vi "Hatch Manipulator Controller.vi"(8 "error in":errorcluster) -> ()   [LabVIEW 2018]
doc: "This VI executes continuously carrying out the current operation and responding to updates or new operations. It will often contain the timing or control code that is difficult to place directly in TeleOp. This VI generally opens all sensors and motors and isolates the rest of the robot code from knowing how the operations are carried out."
uses:
  Hatch Manipulator Setpoints.ctl
  Hatch Manipulator Operations.ctl
  <vilib>/Rock Robotics/WPI/Solenoid/WPI_SolenoidChannel.ctl
  <vilib>/Rock Robotics/WPI/Solenoid/WPI_SolenoidValue.ctl
  <vilib>/Rock Robotics/WPI/Solenoid/WPI_SolenoidOpenSingle.vi
  <vilib>/Rock Robotics/WPI/Solenoid/WPI_SolenoidSetEnum.vi
panel:
  out "Current\nCmd":string
  # "Tip: It may be helpful to observe inputs and sensor values.\nYou may also want to display tuning or debugging controls."
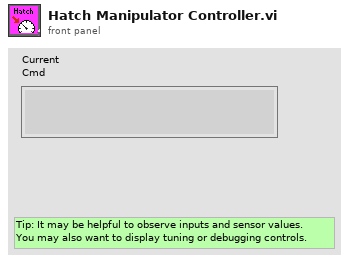
[diagram p1: front panel]
types:
  T1 = typedef "WPI_SolenoidValue.ctl" = enum16{"Off", "On", "Forward", "Reverse"}
  T2 = typedef "WPI_SolenoidChannel.ctl" = enum8{"Solenoid 0", "Solenoid 1", "Solenoid 2", "Solenoid 3", "Solenoid 4", "Solenoid 5", "Solenoid 6", "Solenoid 7", "Invalid"}
  T3 = typedef "Hatch Manipulator Setpoints.ctl" = cluster{"Operation":T4, "Setpoint":dbl, "Duration":dbl}
  T4 = typedef "Hatch Manipulator Operations.ctl" = enum16{"Reserve", "Read Current", "Immediate", "Out", "In", "Open", "Close"}
  T5 = typedef "WPI_SolenoidDevRef.ctl" = cluster{"DevStatus":errorcluster, "Pneumatics Control Module":u8, "Forward Solenoid Channel":T2, "Reverse Solenoid Channel":T2}
  T6 = typedef "Command Status Info.ctl" = cluster{"Name":string, "Status":T7, "notifier out":T8}
  T7 = typedef "Completion Status.ctl" = enum16{"Successful", "Aborted", "Incomplete"}
  T8 = typedef "Completion Notifier.ctl" = refnum<notifier>
  T9 = cluster{"Current Command":T3, "Command Timing":cluster{"Start Time (ms)":u32, "Iterations":i32}, "Command Arguments":cluster{"Command Info":T6, "Description":string, "Default Command":T3, "queue out":refnum<queue>, "Subsystem Name":string}}
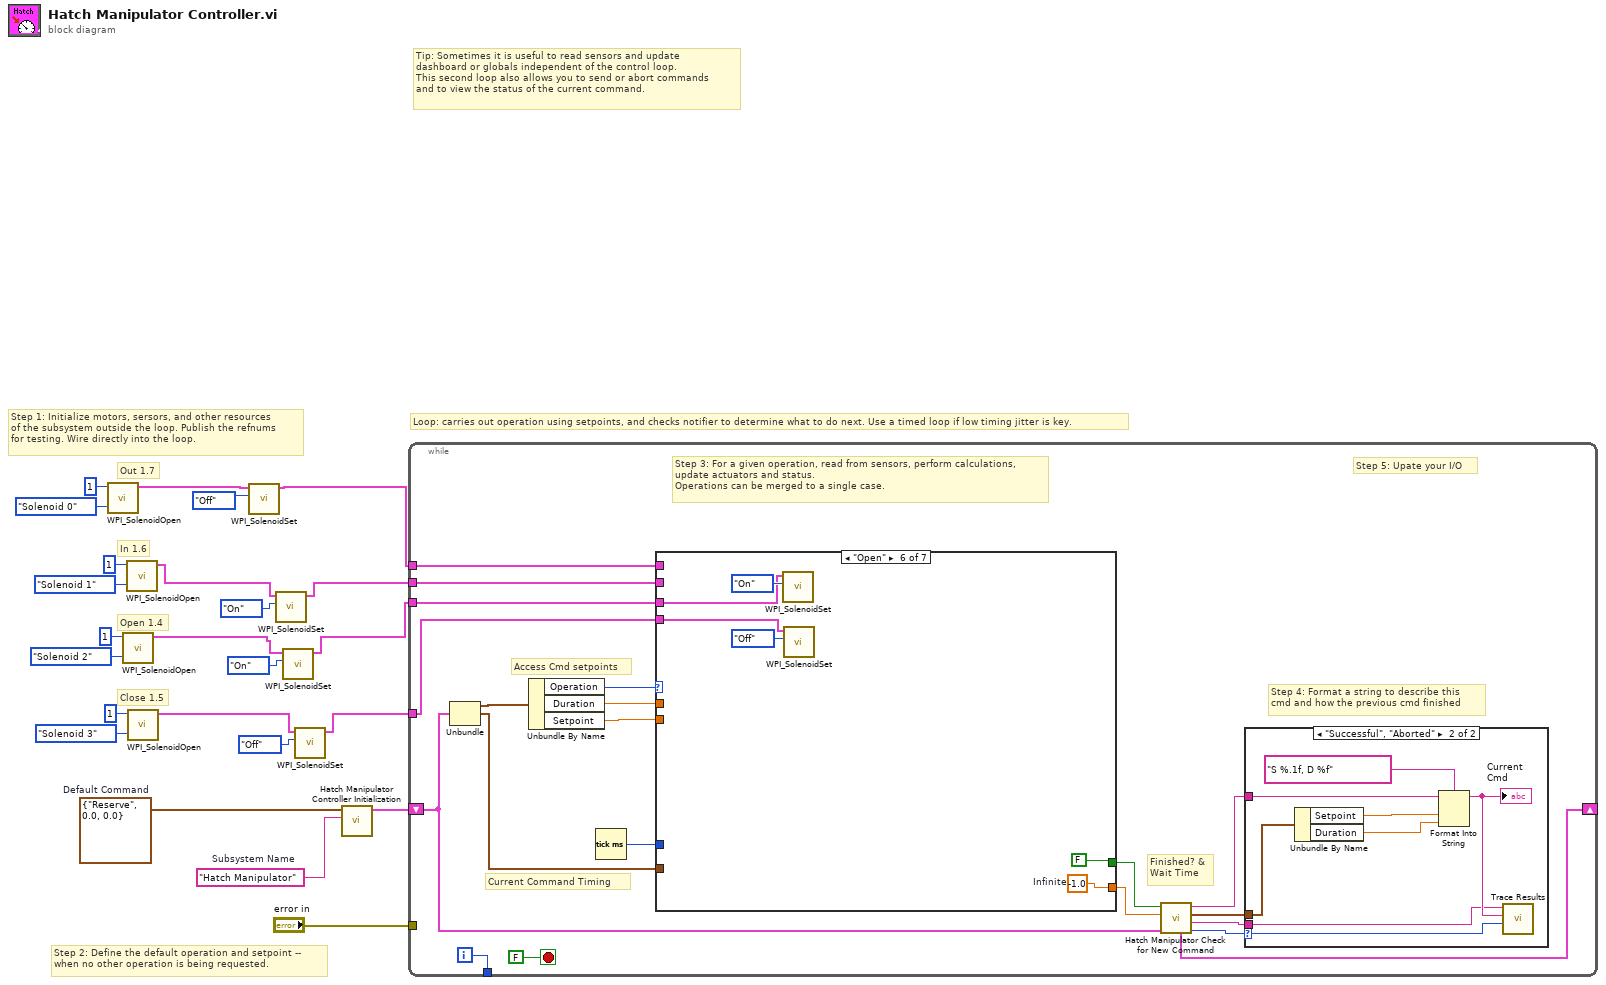
[diagram p0: block diagram]
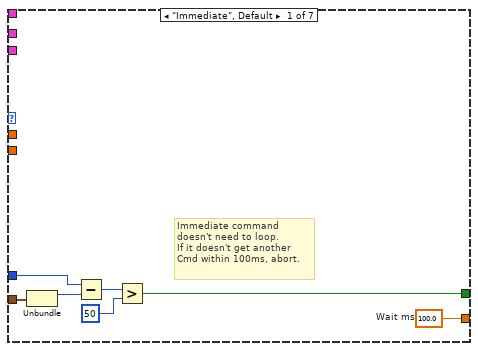
[diagram p3: hidden frame]
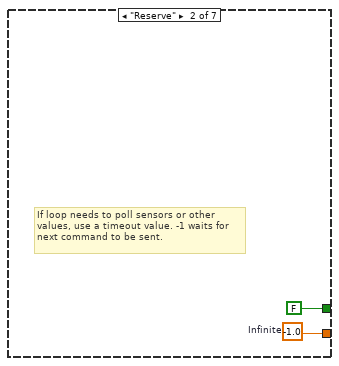
[diagram p4: hidden frame]
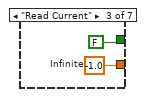
[diagram p5: hidden frame]
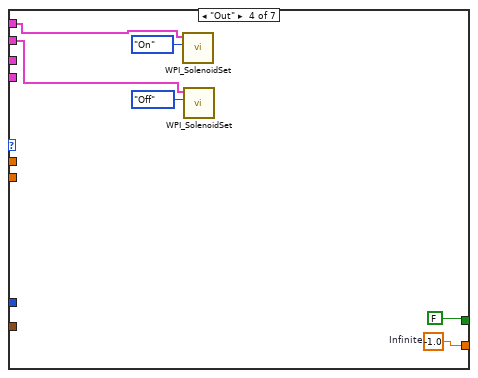
[diagram p6: hidden frame]
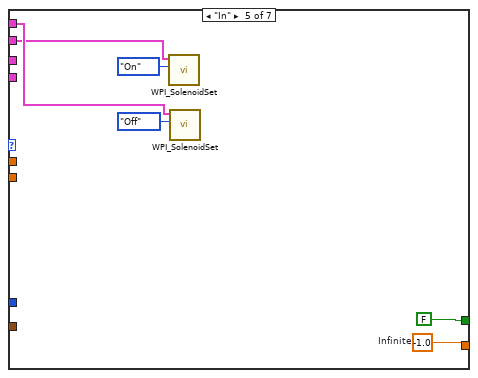
[diagram p7: hidden frame]
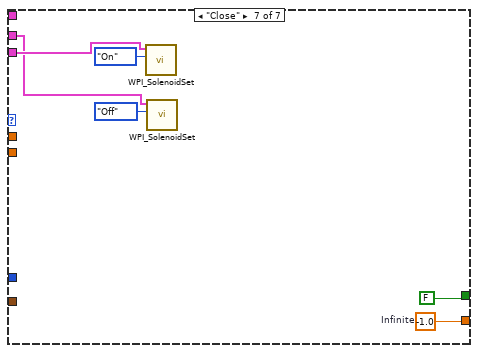
[diagram p8: hidden frame]
diagram:
  w21 = T3 {"Operation"=enum."Reserve", "Setpoint"=0.0, "Duration"=0.0}  # Default Command
  w22 = "Hatch Manipulator"  # Subsystem Name
  # "Close 1.5"
  # "Open 1.4"
  # "In 1.6"
  # "Out 1.7"
  # "Tip: Sometimes it is useful to read sensors and update\ndashboard or globals independent of the control loop.\nThis second loop also allows you to send or abort commands\nand to view the status of the current command."
  # "Step 2: Define the default operation and setpoint --\nwhen no other operation is being requested."
  # "Step 1: Initialize motors, sersors, and other resources\nof the subsystem outside the loop. Publish the refnums\nfor testing. Wire directly into the loop."
  # "Loop: carries out operation using setpoints, and checks notifier to determine what to do next. Use a timed loop if low timing jitter is key."
  n1 = call-poly <vilib>:"WPI_SolenoidOpen.vi"("Solenoid Channel"=WPI_SolenoidChannel."Solenoid 0", "Pneumatics Control Module (0)"=u8 1) -> ("SolenoidDevRef"=w12:T5)  [unwired: 8 in, 1 out]
  n2 = call-poly <vilib>:"WPI_SolenoidOpen.vi"("Solenoid Channel"=WPI_SolenoidChannel."Solenoid 2", "Pneumatics Control Module (0)"=u8 1) -> ("SolenoidDevRef"=w5:T5)  [unwired: 8 in, 1 out]
  n3 = call-poly <vilib>:"WPI_SolenoidOpen.vi"("Solenoid Channel"=WPI_SolenoidChannel."Solenoid 1", "Pneumatics Control Module (0)"=u8 1) -> ("SolenoidDevRef"=w8:T5)  [unwired: 8 in, 1 out]
  n4 = call-poly <vilib>:"WPI_SolenoidOpen.vi"("Solenoid Channel"=WPI_SolenoidChannel."Solenoid 3", "Pneumatics Control Module (0)"=u8 1) -> ("SolenoidDevRef"=w2:T5)  [unwired: 8 in, 1 out]
  n5 = call-poly <vilib>:"WPI_SolenoidSet.vi"("Value"=WPI_SolenoidValue."Off", "SolenoidDevRef"=w12) -> ("SolenoidDevRef"=w11:T5)  [unwired: 8 in, 1 out]
  n6 = call-poly <vilib>:"WPI_SolenoidSet.vi"("Value"=WPI_SolenoidValue."On", "SolenoidDevRef"=w8) -> ("SolenoidDevRef"=w7:T5)  [unwired: 8 in, 1 out]
  n7 = call-poly <vilib>:"WPI_SolenoidSet.vi"("Value"=WPI_SolenoidValue."On", "SolenoidDevRef"=w5) -> ("SolenoidDevRef"=w4:T5)  [unwired: 8 in, 1 out]
  n8 = call-poly <vilib>:"WPI_SolenoidSet.vi"("Value"=WPI_SolenoidValue."Off", "SolenoidDevRef"=w2) -> ("SolenoidDevRef"=w1:T5)  [unwired: 8 in, 1 out]
  n9 = call "Hatch Manipulator Controller Initialization.vi"("Subsystem Name"=w22, "Default Command"=w21) -> ("Current Command"=w23:T9)  [unwired: 9 in]
  n10 = while {
    shift-right: [w36] -> _
    shift-left: w23 -> [w29]
    tunnel: [w43] -> _
    tunnel: "error in" -> [_]
    tunnel: w11 -> [w28]
    tunnel: w7 -> [w27]
    tunnel: w4 -> [w26]
    tunnel: w1 -> [w25]
    i -> [w43]
    stop <- FALSE stop-if-true
    # "Step 5: Upate your I/O"
    # "Step 4: Format a string to describe this\ncmd and how the previous cmd finished"
    # "Current Command Timing"
    # "Access Cmd setpoints"
    # "Finished? &\nWait Time"
    # "Step 3: For a given operation, read from sensors, perform calculations,\nupdate actuators and status.\nOperations can be merged to a single case."
    n11 = Unbundle(w29) -> ("Current Command"=w42:T3, "Command Timing"=w38:cluster{"Start Time (ms)":u32, "Iterations":i32})  [unwired: 1 out]
    n12 = Unbundle By Name(w42) -> ("Operation"=w41:T4, "Duration"=w40:dbl, "Setpoint"=w37:dbl)
    n13 = Tick Count (ms)() -> (millisecond timer value=w39:u32)
    n14 = case shown="\"Open\"" w41 {
      tunnel: [w59 w61 w62 w64 w70 w76 w82] -> w34
      tunnel: [w53 FALSE ("ignore previous (F)") FALSE ("ignore previous (F)") FALSE ("ignore previous (F)") FALSE ("ignore previous (F)") FALSE ("ignore previous (F)") FALSE ("ignore previous (F)")] -> w35
      tunnel: w38 -> [w55 _ _ _ _ _ _]
      tunnel: w40 -> [_ _ _ _ _ _ _]
      tunnel: w39 -> [w54 _ _ _ _ _ _]
      tunnel: w37 -> [_ _ _ _ _ _ _]
      tunnel: w28 -> [_ _ _ w67 w73 _ _]
      tunnel: w27 -> [_ _ _ w66 w72 _ _]
      tunnel: w26 -> [_ _ _ _ _ w79 w84]
      tunnel: w25 -> [_ _ _ _ _ w78 w85]
      frame "Immediate", Default {
        w59 = 100.0  # Wait ms
        # "Immediate command\ndoesn't need to loop.\nIf it doesn't get another\nCmd within 100ms, abort."
        n15 = Unbundle(w55) -> ("Start Time (ms)"=w58:u32)  [unwired: 1 out]
        n16 = Subtract(x=w54, y=w58) -> (x-y=w57:u32)
        n17 = Greater?(x=w57, y=u8 50 ("Left Motor")) -> (0:w53:bool)
      }
      frame "Reserve" {
        w61 = -1.0  # Infinite
        # "If loop needs to poll sensors or other\nvalues, use a timeout value. -1 waits for\nnext command to be sent."
      }
      frame "Read Current" {
        w62 = -1.0  # Infinite
      }
      frame "Out" {
        w64 = -1.0  # Infinite
        n18 = call-poly <vilib>:"WPI_SolenoidSet.vi"("Value"=WPI_SolenoidValue."On", "SolenoidDevRef"=w67) -> ()  [unwired: 8 in, 2 out]
        n19 = call-poly <vilib>:"WPI_SolenoidSet.vi"("Value"=WPI_SolenoidValue."Off", "SolenoidDevRef"=w66) -> ()  [unwired: 8 in, 2 out]
      }
      frame "In" {
        w70 = -1.0  # Infinite
        n20 = call-poly <vilib>:"WPI_SolenoidSet.vi"("Value"=WPI_SolenoidValue."On", "SolenoidDevRef"=w72) -> ()  [unwired: 8 in, 2 out]
        n21 = call-poly <vilib>:"WPI_SolenoidSet.vi"("Value"=WPI_SolenoidValue."Off", "SolenoidDevRef"=w73) -> ()  [unwired: 8 in, 2 out]
      }
      frame "Open" {
        w76 = -1.0  # Infinite
        n22 = call-poly <vilib>:"WPI_SolenoidSet.vi"("Value"=WPI_SolenoidValue."On", "SolenoidDevRef"=w79) -> ()  [unwired: 8 in, 2 out]
        n23 = call-poly <vilib>:"WPI_SolenoidSet.vi"("Value"=WPI_SolenoidValue."Off", "SolenoidDevRef"=w78) -> ()  [unwired: 8 in, 2 out]
      }
      frame "Close" {
        w82 = -1.0  # Infinite
        n24 = call-poly <vilib>:"WPI_SolenoidSet.vi"("Value"=WPI_SolenoidValue."On", "SolenoidDevRef"=w85) -> ()  [unwired: 8 in, 2 out]
        n25 = call-poly <vilib>:"WPI_SolenoidSet.vi"("Value"=WPI_SolenoidValue."Off", "SolenoidDevRef"=w84) -> ()  [unwired: 8 in, 2 out]
      }
    }
    n26 = call "Hatch Manipulator Check for New Command.vi"("Current Command"=w29, "Wait time (ms)"=w34, "Finished?"=w35) -> ("Completion"=w30:T7, "Subsystem Name"=w31:string, "Current Command"=w32:T3, "Initial Trace String"=w33:string, "NextCommand"=w36:T9)  [unwired: 4 in]
    n27 = case shown="\"Successful\", \"Aborted\"" w30 {
      selector: w30 -> [_ w52]
      tunnel: w33 -> [_ w48]
      tunnel: w32 -> [_ w49]
      tunnel: w31 -> [_ w45]
      frame "Incomplete", Default {
        # "Continuing current command"
      }
      frame "Successful", "Aborted" {
        # "Report and setup for next command"
        n28 = Unbundle By Name(w49) -> ("Setpoint"=w51:dbl, "Duration"=w46:dbl)
        n29 = Format Into String(format string="S %.1f, D %f", initial string=w48, w51, w46) -> (resulting string=w47:string)  [unwired: 1 in, 1 out]
        "Current\nCmd" <- w47
        n30 = call <vilib>:"Trace Results.vi"("Status of previous command"=w52, "Description"=w47, "Subsystem"=w45) -> ()  [unwired: 9 in]
      }
    }
  }
